vi "Teardown.vi"(8 "Error In":errorcluster, 11 "File Info":refnum<class "File Info.lvclass">) -> (0 "Error Out":errorcluster)   [LabVIEW 2018, in "Tests.lvlib" / "File Info.lvlib"]
uses:
  File Info.lvlib
  src/Toolkit/File Info/File Info.lvclass
  src/Toolkit/File Info/Support/Destroy to SSH.vi
  src/Toolkit/SSH/SSH.lvclass
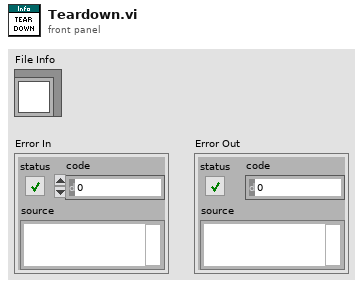
[diagram p1: front panel]
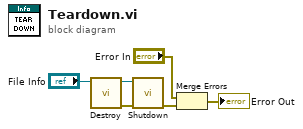
[diagram p0: block diagram]
diagram:
  n1 = call-poly "Destroy.vi"("File Info"="File Info") -> ("Error Out"=w2:errorcluster, "SSH"=w3:refnum<class "SSH.lvclass">)  [unwired: 9 in]
  n2 = call "Shutdown.vi"("Error In"=w2, "SSH"=w3) -> ("Error Out"=w6:errorcluster)  [unwired: 9 in]
  n3 = Merge Errors("Error In", w6) -> (→"Error Out":errorcluster)
